vi "comms_BT_Open.vi"(8 "error in (no error)":errorcluster, 9 "BT uuid":string, 10 "BT Channel (0)":u16, 11 "BT address":string) -> (0 "error out":errorcluster, 2 "Response":string, 3 "Bluetooth Network Connection out":refnum<k31>)   [LabVIEW 2018]
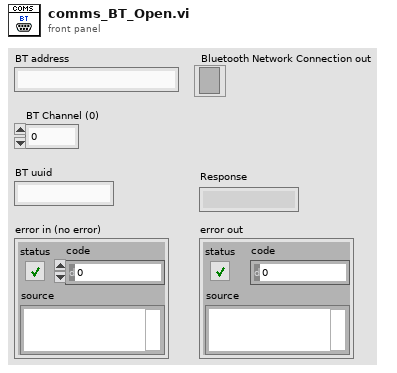
[diagram p1: front panel]
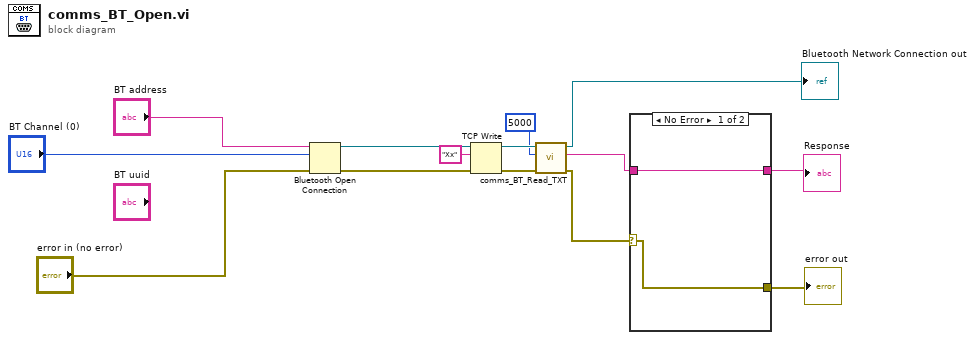
[diagram p0: block diagram]
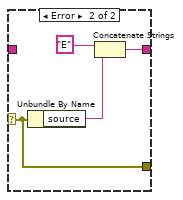
[diagram p2: hidden frame]
diagram:
  n1 = Bluetooth Open Connection(8:"error in (no error)", 10:"BT Channel (0)", 11:"BT address") -> (0:w3:errorcluster, 3:w11:refnum<k31>)  [unwired: 2 in]
  n2 = TCP Write(connection ID=w11, data in="Xx", error in (no error)=w3) -> (connection ID out=w9:refnum<k31>, error out=w8:errorcluster)  [unwired: 1 in, 1 out]
  n3 = call "comms_BT_Read_TXT.vi"("error in"=w8, "timeout ms (25000)"=5000, "connection ID"=w9) -> ("error out"=w6:errorcluster, "Data Out"=w7:string, "connection ID Out"=→"Bluetooth Network Connection out":refnum<k31>)  [unwired: 5 in, 1 out]
  n4 = case shown="No Error" w6 {
    selector: w6 -> [w16 w20]
    tunnel: [w16 w20] -> w2
    tunnel: w7 -> [w15 _]
    tunnel: [w15 w19] -> w4
    frame No Error {
    }
    frame Error {
      n5 = Unbundle By Name(w20) -> ("source"=w18:string)
      n6 = Concatenate Strings("E", w18) -> (w19:string)
    }
  }
  "error out" <- w2
  "Response" <- w4
